vi "Configure Channel (Volt Delta).vi"(0 "VISA resource name":refnum<visa-resource-name>, 1 "Reference Channel (0001)":string="0001", 5 "Channel (0001)":string="0001", 7 "Enable Channel (True)":bool=TRUE, 9 "Range And Span":T1={"Volt Range (4 : 2V)"=4, "Enable Span (False)"=FALSE, "Lower Span (-2.0000)"=-2.0, "Upper Span (2.0000)"=2.0, "Bias (0)"=0.0} {"Upper Span (2.0000)" min=-99999.0 max=99999.0 step=1.0 format="%_5g"; "Lower Span (-2.0000)" min=-99999.0 max=99999.0 step=1.0 format="%_5g"; "Volt Range (4 : 2V)" items=["20mV", "60mV", "200mV", "1V", "2V", "6V", "20V", "50V"]}, 11 "error in (no error)":errorcluster) -> (4 "VISA resource name out":refnum<visa-resource-name>, 6 "Channel":string, 15 "error out":errorcluster)   [LabVIEW 2020, in "Yokogawa GX Series.lvlib"]
doc: "Sets the input range as voltage.\n\nCommand: SRangeAI"
uses:
  <instrlib>/Yokogawa GX Series/Yokogawa GX Series.lvlib
  <instrlib>/Yokogawa GX Series/Private/Volt Range.vi
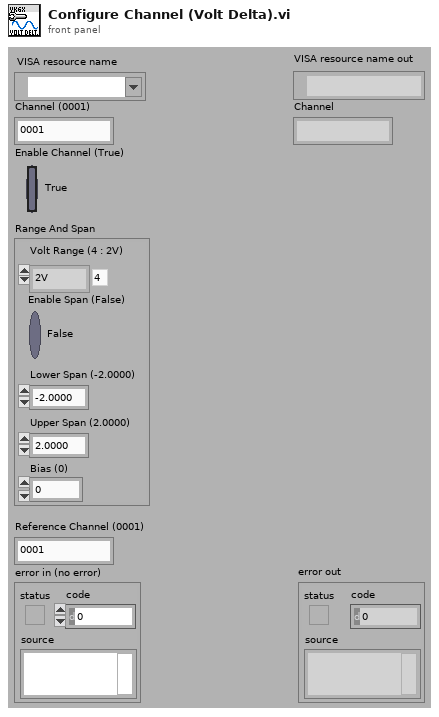
[diagram p1: front panel]
types:
  T1 = cluster{"Volt Range (4 : 2V)":i32, "Enable Span (False)":bool, "Lower Span (-2.0000)":dbl, "Upper Span (2.0000)":dbl, "Bias (0)":dbl}
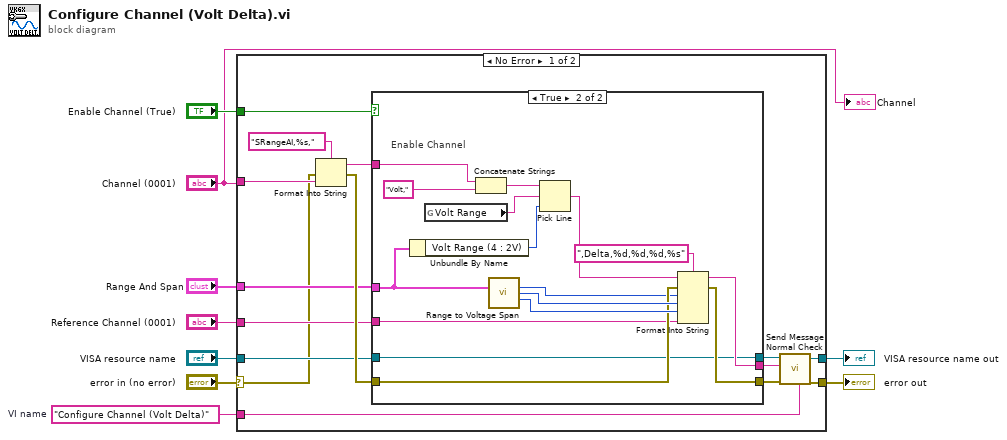
[diagram p0: block diagram]
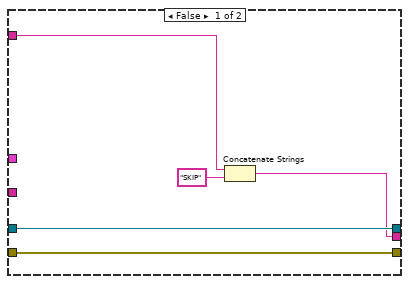
[diagram p2: hidden frame]
diagram:
  w5 = "Configure Channel (Volt Delta)"  # VI name
  n1 = case shown="No Error" "error in (no error)" {
    selector: "error in (no error)" -> [w10 w46]
    tunnel: "Enable Channel (True)" -> [w21 _]
    tunnel: "VISA resource name" -> [w20 w47]
    tunnel: [w18 w47] -> w7
    tunnel: [w17 w46] -> w6
    tunnel: w5 -> [w14 _]
    tunnel: "Range And Span" -> [w13 _]
    tunnel: "Reference Channel (0001)" -> [w12 _]
    tunnel: "Channel (0001)" -> [w11 _]
    frame No Error {
      n2 = Format Into String(format string="SRangeAI,%s,", error in=w10, w11) -> (resulting string=w22:string, error out=w23:errorcluster)  [unwired: 1 in]
      n3 = case shown="True" w21 {
        tunnel: w23 -> [w28 w36]
        tunnel: w12 -> [_ w32]
        tunnel: [w28 w41] -> w19
        tunnel: w22 -> [w29 w43]
        tunnel: w20 -> [w26 w34]
        tunnel: [w26 w34] -> w15
        tunnel: [w25 w40] -> w16
        tunnel: w13 -> [_ w33]
        frame False {
          n4 = Concatenate Strings(w29, "SKIP") -> (w25:string)
        }
        frame True {
          # "Enable Channel"
          n5 = Unbundle By Name(w33) -> ("Volt Range (4 : 2V)"=w39:i32)
          n6 = global read "Volt Range.vi" "Volt Range"() -> (w30:string)
          n7 = Concatenate Strings(w43, "Volt,") -> (w42:string)
          n8 = call <instrlib>:"Range to Voltage Span.vi"("Range And Span"=w33) -> ("Lower Span"=w35:i32, "Upper Span"=w38:i32, "Bias"=w37:i32)  [unwired: 8 in, 4 out]
          n9 = Pick Line(string ("")=w42, multi-line string=w30, line index=w39) -> (output string=w44:string)
          n10 = Format Into String(format string=",Delta,%d,%d,%d,%s", initial string=w44, error in=w36, w35, w38, w37, w32) -> (resulting string=w40:string, error out=w41:errorcluster)
        }
      }
      n11 = call <instrlib>:"Send Message Normal Check.vi"("Source (\"\")"=w14, "error in (no error)"=w19, "Send Message (\"\")"=w16, "VISA resource name"=w15) -> ("error out"=w17:errorcluster, "VISA resource name out"=w18:refnum<visa-resource-name>)  [unwired: 2 in, 4 out]
    }
    frame Error {
    }
  }
  "error out" <- w6
  "VISA resource name out" <- w7
  "Channel" <- "Channel (0001)"
